vi "Easy_action.vi"() -> ()   [LabVIEW 2016]
uses:
  Classes/Controllers/Motion/Copy of Motion Folder/Motion.lvclass
  Classes/Controllers/Camera/Copy of Controller Folder/Controller.lvclass
panel:
  in  "Array":dbl[](array[numeric])
  in  "go":bool
  in  "stop":bool
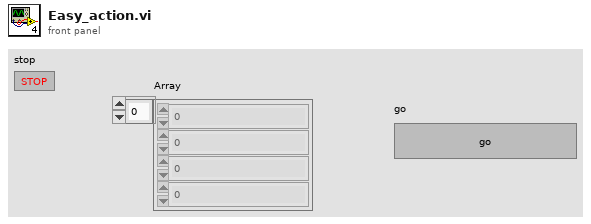
[diagram p1: front panel]
types:
  T1 = typedef "Controller.lvclass/Controllers.ctl" = cluster{"Copy of Motion.lvclass":refnum<class "Motion.lvclass">, "Copy of I-O.lvclass":refnum<class "I-O.lvclass">, "Copy of Dispenser.lvclass":refnum<class "Dispenser.lvclass">}
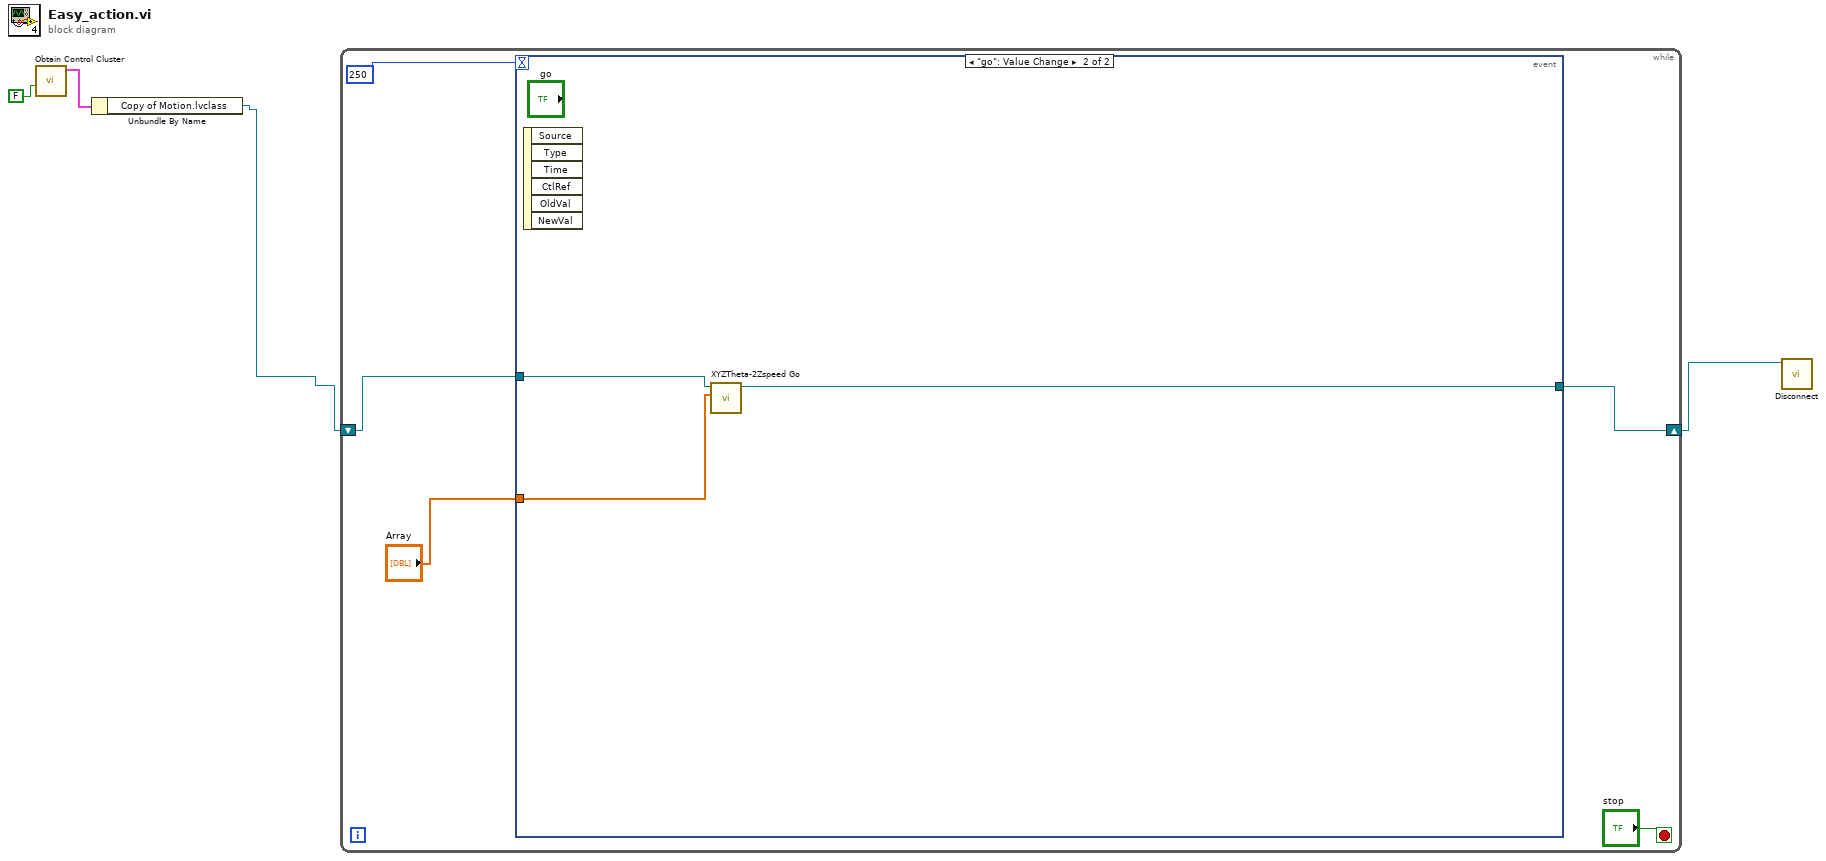
[diagram p0: block diagram]
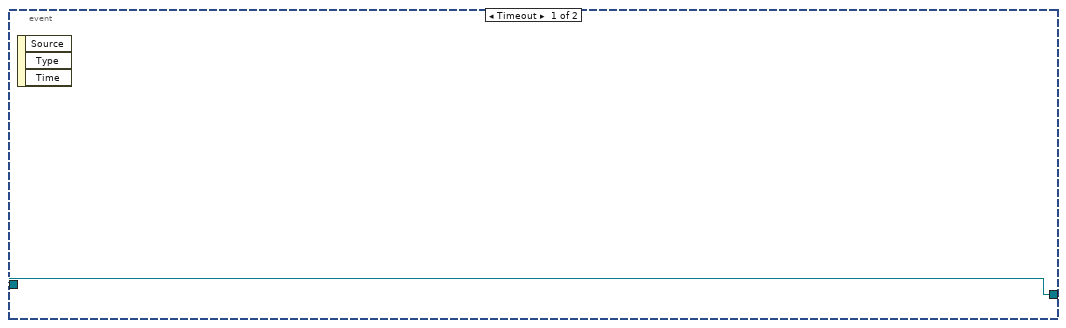
[diagram p2: hidden frame]
diagram:
  n1 = call "Obtain Control Cluster.vi"("I/O"=FALSE) -> ("Control Out"=w3:T1)  [unwired: 10 in]
  n2 = Unbundle By Name(w3) -> ("Copy of Motion.lvclass"=w2:refnum<class "Motion.lvclass">)
  n3 = while {
    shift-right: [w7] -> w1
    shift-left: w2 -> [w6]
    stop <- "stop" stop-if-true
    n4 = event shown="[1] \"go\": Value Change" {
      selector: _ -> [_ _]
      dyn-events: _ -> [_ _]
      timeout: 250 -> [_ _]
      tunnel: w6 -> [w10 w13]
      tunnel: [w10 w12] -> w7
      tunnel: "Array" -> [_ w11]
      event Timeout {
        n5 = event-data() -> ()  [unwired: 1 in, 3 out]
      }
      event "go": Value Change {
        n6 = event-data() -> ()  [unwired: 1 in, 6 out]
        n7 = call "XYZTheta-2Zspeed Go.vi"("XYZTheta In"=w11, "Motion in"=w13) -> ("Motion out"=w12:refnum<class "Motion.lvclass">)  [unwired: 7 in, 2 out]
      }
    }
  }
  n8 = call-dynamic "Disconnect.vi"("Controller in"=w1) -> ()  [unwired: 9 in, 1 out]
